vi "Gate Delay Queue Engine 01.vi"   [LabVIEW 2016]
uses:
  Gate Delay Type Defs/Gate Delay Notifier Element.ctl
  Gate Delay Type Defs/Gate Delay Actions.ctl
  <vilib>/Instr/_visa.llb/VISA Configure Serial Port (Instr).vi
types:
  T1 = typedef "Gate Delay Notifier Element.ctl" = cluster{"Gate Delay Actions":T2, "Laser Delay":dbl, "Window Delay":dbl, "Window Width":dbl, "Command Received?":bool}
  T2 = typedef "Gate Delay Actions.ctl" = enum16{"Set Laser Delay", "Set Window Delay", "Set Window Width", "Get Delays", "Set Default Delays", "Restore Defaults", "Quit"}
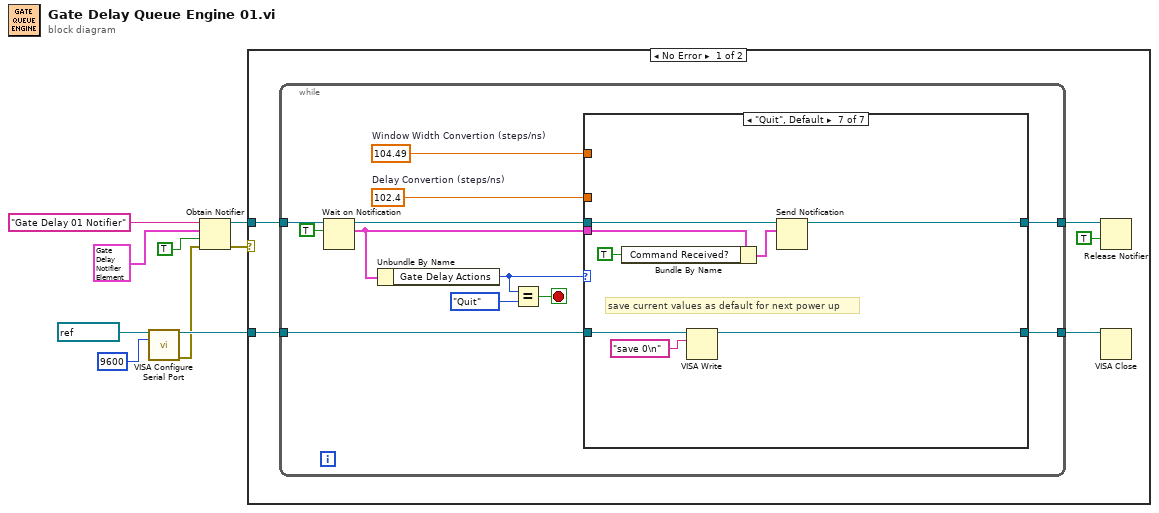
[diagram p0: block diagram]
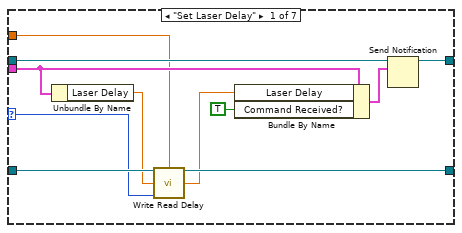
[diagram p2: hidden frame]
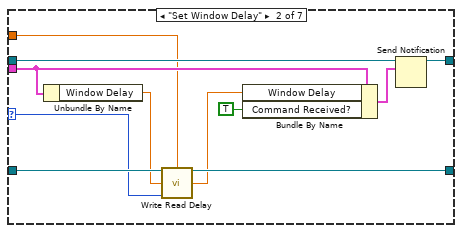
[diagram p3: hidden frame]
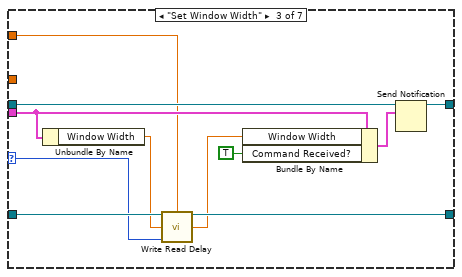
[diagram p4: hidden frame]
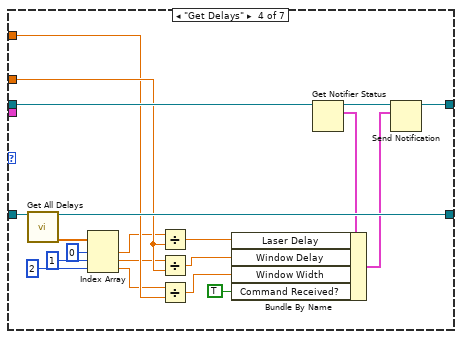
[diagram p5: hidden frame]
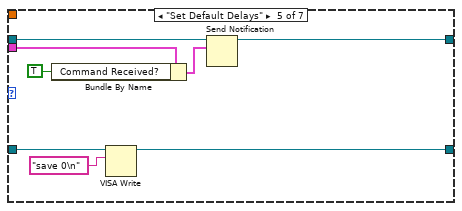
[diagram p6: hidden frame]
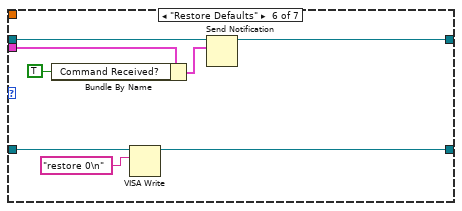
[diagram p7: hidden frame]
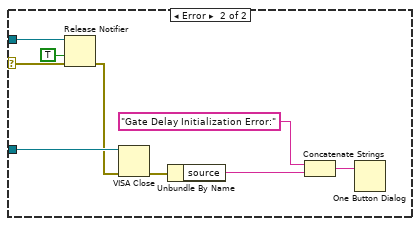
[diagram p8: hidden frame]
diagram:
  n1 = call-poly "VISA Configure Serial Port"("VISA resource name"=refnum<visa-resource-name> "COM3", "baud rate (9600)"=u32 9600) -> ("VISA resource name out"=w4:refnum<visa-resource-name>, "error out"=w3:errorcluster)  [unwired: 12 in]
  n2 = Obtain Notifier(name (unnamed)="Gate Delay 01 Notifier", notification data type=T1 {"Gate Delay Actions"=enum."Set Laser Delay", "Laser Delay"=0.0, "Window Delay"=0.0, "Window Width"=0.0, "Command Received?"=FALSE} ("Gate Delay Notifier Element"), create if not found? (T)=TRUE, error in (no error)=w3) -> (notifier out=w6:refnum<notifier>, error out=w2:errorcluster)  [unwired: 1 out]
  n3 = case shown="No Error" w2 {
    selector: w2 -> [_ w104]
    tunnel: w6 -> [w13 w112]
    tunnel: w4 -> [w14 w107]
    frame No Error {
      n4 = while {
        tunnel: w14 -> [w22]
        tunnel: w13 -> [w20]
        tunnel: [w21] -> w12
        tunnel: [w17] -> w11
        stop <- w25 stop-if-true
        w24 = 102.4  # Delay Convertion (steps/ns)
        w23 = 104.49  # Window Width Convertion (steps/ns)
        n5 = Wait on Notification(notifier=w20, ignore previous (F)=TRUE) -> (notifier out=w19:refnum<notifier>, notification=w16:T1)  [unwired: 2 in, 2 out]
        n6 = Unbundle By Name(w16) -> ("Gate Delay Actions"=w18:T2)
        n7 = Equal?(x=w18, y=Gate_Delay_Actions."Quit") -> (x = y?=w25:bool)
        n8 = case shown="\"Quit\", Default" w18 {
          selector: w18 -> [w29 w40 w51 _ _ _ _]
          tunnel: w24 -> [w27 w38 _ w68 _ _ _]
          tunnel: w23 -> [_ _ w49 w64 _ _ _]
          tunnel: w22 -> [w32 w43 w54 w79 w81 w89 w103]
          tunnel: w19 -> [w36 w47 w58 w78 w85 w93 w98]
          tunnel: [w31 w42 w53 w76 w80 w88 w102] -> w21
          tunnel: [w35 w46 w57 w73 w83 w91 w96] -> w17
          tunnel: w16 -> [w33 w44 w55 _ w87 w95 w97]
          frame "Set Laser Delay" {
            n9 = Unbundle By Name(w33) -> ("Laser Delay"=w30:dbl)
            n10 = call "Write Read Delay.vi"("Visa Ref"=w32, "Conversion (steps/ns)"=w27, "Delay (ns)"=w30, "Gate Delay Actions"=w29) -> ("Visa Ref Dup"=w31:refnum<visa-resource-name>, "Delay Out (ns)"=w28:dbl)  [unwired: 10 in]
            n11 = Bundle By Name(cluster=w33, "Laser Delay"=w28, "Command Received?"=TRUE) -> (w34:T1)
            n12 = Send Notification(notification=w34, notifier=w36) -> (notifier out=w35:refnum<notifier>)  [unwired: 1 in, 1 out]
          }
          frame "Set Window Delay" {
            n13 = Unbundle By Name(w44) -> ("Window Delay"=w41:dbl)
            n14 = call "Write Read Delay.vi"("Visa Ref"=w43, "Conversion (steps/ns)"=w38, "Delay (ns)"=w41, "Gate Delay Actions"=w40) -> ("Visa Ref Dup"=w42:refnum<visa-resource-name>, "Delay Out (ns)"=w39:dbl)  [unwired: 10 in]
            n15 = Bundle By Name(cluster=w44, "Window Delay"=w39, "Command Received?"=TRUE) -> (w45:T1)
            n16 = Send Notification(notification=w45, notifier=w47) -> (notifier out=w46:refnum<notifier>)  [unwired: 1 in, 1 out]
          }
          frame "Set Window Width" {
            n17 = Unbundle By Name(w55) -> ("Window Width"=w52:dbl)
            n18 = call "Write Read Delay.vi"("Visa Ref"=w54, "Conversion (steps/ns)"=w49, "Delay (ns)"=w52, "Gate Delay Actions"=w51) -> ("Visa Ref Dup"=w53:refnum<visa-resource-name>, "Delay Out (ns)"=w50:dbl)  [unwired: 10 in]
            n19 = Bundle By Name(cluster=w55, "Window Width"=w50, "Command Received?"=TRUE) -> (w56:T1)
            n20 = Send Notification(notification=w56, notifier=w58) -> (notifier out=w57:refnum<notifier>)  [unwired: 1 in, 1 out]
          }
          frame "Get Delays" {
            n21 = call "Get All Delays.vi"("VISA Ref"=w79) -> ("VISA Ref Dup"=w76:refnum<visa-resource-name>, "Delays (steps)"=w72:dbl[])  [unwired: 13 in]
            n22 = Index Array(array=w72, index #1=0 ("index"), index #2=1 ("index"), index #3=2 ("index")) -> (element #1=w62:dbl, element #2=w60:dbl, element #3=w61:dbl)
            n23 = Divide(x=w62, y=w68) -> (x/y=w67:dbl)
            n24 = Divide(x=w60, y=w68) -> (x/y=w66:dbl)
            n25 = Divide(x=w61, y=w64) -> (x/y=w65:dbl)
            n26 = Get Notifier Status(notifier=w78) -> (notifier out=w77:refnum<notifier>, current notification=w75:T1)  [unwired: 1 in, 3 out]
            n27 = Bundle By Name(cluster=w75, "Laser Delay"=w67, "Window Delay"=w66, "Window Width"=w65, "Command Received?"=TRUE) -> (w74:T1)
            n28 = Send Notification(notification=w74, notifier=w77) -> (notifier out=w73:refnum<notifier>)  [unwired: 1 in, 1 out]
          }
          frame "Set Default Delays" {
            n29 = Bundle By Name(cluster=w87, "Command Received?"=TRUE) -> (w84:T1)
            n30 = VISA Write(VISA resource name=w81, write buffer="save 0\n") -> (VISA resource name out=w80:refnum<visa-resource-name>)  [unwired: 1 in, 2 out]
            n31 = Send Notification(notification=w84, notifier=w85) -> (notifier out=w83:refnum<notifier>)  [unwired: 1 in, 1 out]
          }
          frame "Restore Defaults" {
            n32 = Bundle By Name(cluster=w95, "Command Received?"=TRUE) -> (w92:T1)
            n33 = VISA Write(VISA resource name=w89, write buffer="restore 0\n") -> (VISA resource name out=w88:refnum<visa-resource-name>)  [unwired: 1 in, 2 out]
            n34 = Send Notification(notification=w92, notifier=w93) -> (notifier out=w91:refnum<notifier>)  [unwired: 1 in, 1 out]
          }
          frame "Quit", Default {
            # "save current values as default for next power up"
            n35 = Bundle By Name(cluster=w97, "Command Received?"=TRUE) -> (w100:T1)
            n36 = VISA Write(VISA resource name=w103, write buffer="save 0\n") -> (VISA resource name out=w102:refnum<visa-resource-name>)  [unwired: 1 in, 2 out]
            n37 = Send Notification(notification=w100, notifier=w98) -> (notifier out=w96:refnum<notifier>)  [unwired: 1 in, 1 out]
          }
        }
      }
      n38 = Release Notifier(notifier=w11, force destroy? (F)=TRUE) -> ()  [unwired: 1 in, 3 out]
      n39 = VISA Close(VISA resource name=w12) -> ()  [unwired: 1 in, 1 out]
    }
    frame Error {
      n40 = Release Notifier(notifier=w112, force destroy? (F)=TRUE, error in (no error)=w104) -> (error out=w106:errorcluster)  [unwired: 2 out]
      n41 = VISA Close(VISA resource name=w107, error in (no error)=w106) -> (error out=w105:errorcluster)
      n42 = Unbundle By Name(w105) -> ("source"=w110:string)
      n43 = Concatenate Strings("Gate Delay Initialization Error:", w110) -> (w108:string)
      n44 = One Button Dialog(message=w108) -> ()  [unwired: 1 in, 1 out]
    }
  }
